vi "example-tx-c_api.vi"() -> ()   [LabVIEW 2024]
uses:
  <vilib>/Analysis/1siggen.llb/Ramp Pattern by Samples.vi
  uhd (generated from wizard into user.lib - manually fixed for rx example)/uhd.lvlib
  <vilib>/Analysis/NI_AALBase.lvlib
panel:
  out "ant_out out":string
  in  "stop":bool
  out "freq_out out":dbl
  in  "target_freq":dbl=1000000000.0 format="%#_6p"
  in  "ant":string="TX/RX"
  out "gain_out out":dbl
  in  "gain":dbl
  out "rate_out out":dbl
  in  "rate":dbl=1000000.0
  in  "chan":u64
  out "error out":errorcluster
  in  "args":string="type=b200"
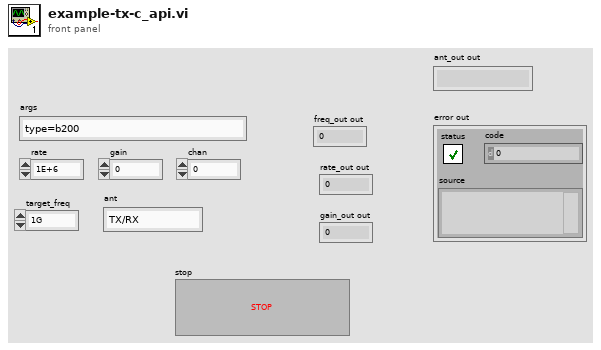
[diagram p1: front panel]
types:
  T1 = cluster{"cpu_format":string, "otw_format":string, "args":string, "channel_list":u64[], "n_channels":u64}
  T2 = cluster{"target_freq":dbl, "rf_freq_policy":u32, "@dummy control@":i8, "@dummy control@":i8, "@dummy control@":i8, "@dummy control@":i8, "rf_freq":dbl, "dsp_freq_policy":u32, "@dummy control@":i8, "@dummy control@":i8, "@dummy control@":i8, "@dummy control@":i8, "dsp_freq":dbl, "args":u64}
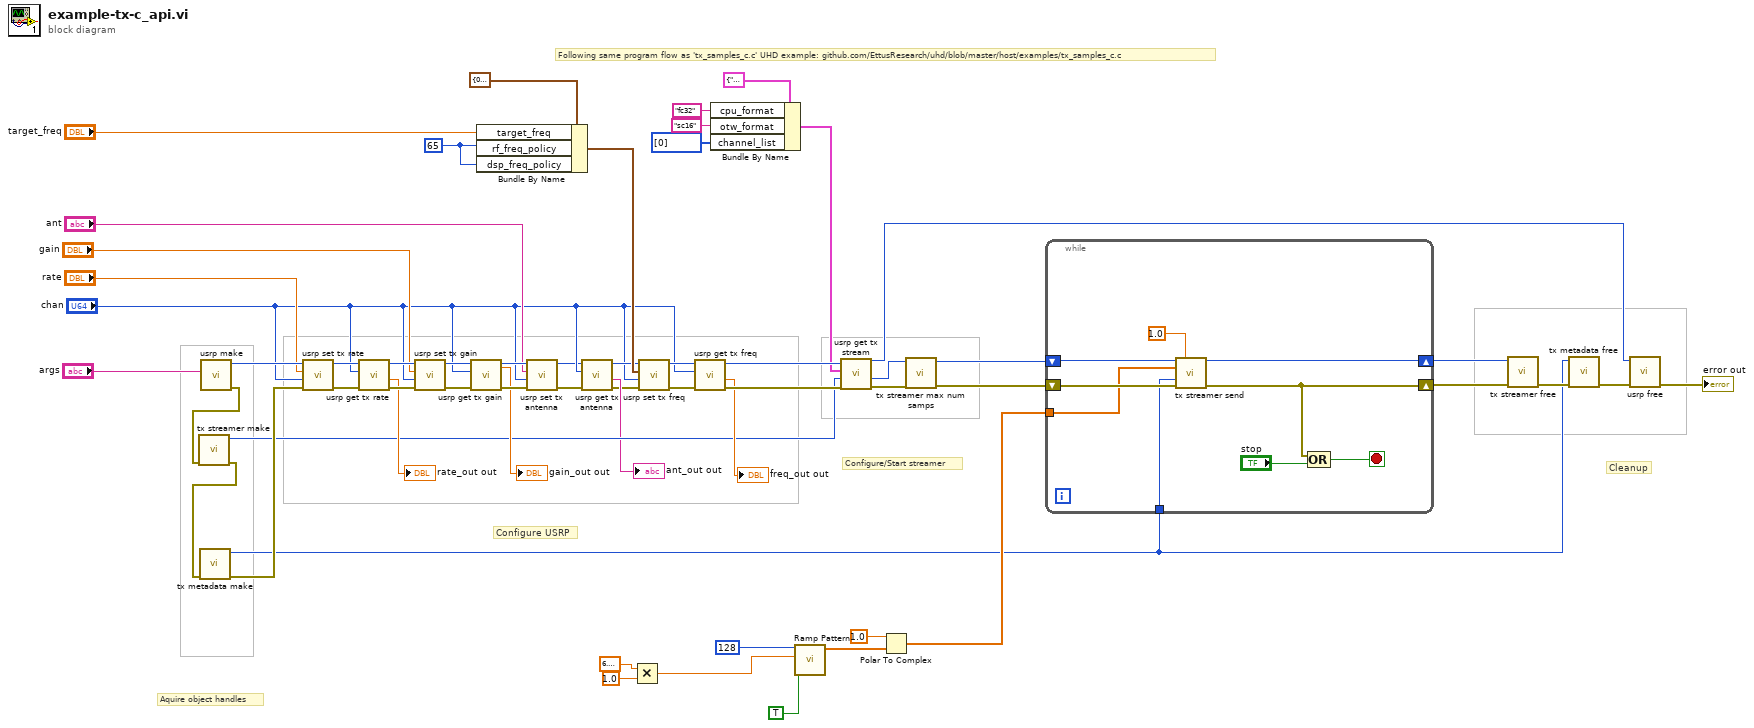
[diagram p0: block diagram]
diagram:
  w16 = u32 65 ("rf_freq_policy")
  # "Cleanup"
  # "Configure/Start streamer"
  # "Configure USRP"
  # "Aquire object handles"
  # "Following same program flow as 'tx_samples_c.c' UHD example: github.com/EttusResearch/uhd/blob/master/host/examples/tx_samples_c.c"
  n1 = call "usrp make.vi"("args"="args") -> ("error out"=w58:errorcluster, "h"=w56:u64)  [unwired: 8 in, 1 out]
  n2 = call "tx streamer make.vi"("error in (no error)"=w58) -> ("error out"=w42:errorcluster, "h out"=w13:u64)  [unwired: 8 in, 1 out]
  n3 = call "tx metadata make.vi"("error in (no error)"=w42) -> ("error out"=w55:errorcluster, "handle out"=w7:u64)  [unwired: 8 in, 1 out]
  n4 = call "usrp set tx rate.vi"("error in (no error)"=w55, "chan"="chan", "rate"="rate", "h"=w56) -> ("error out"=w54:errorcluster, "h 2"=w41:u64)  [unwired: 5 in, 1 out]
  n5 = call "usrp get tx rate.vi"("error in (no error)"=w54, "chan"="chan", "h"=w41) -> ("error out"=w53:errorcluster, "rate_out out"=→"rate_out out":dbl, "h 2"=w40:u64)  [unwired: 5 in, 1 out]
  n6 = call "usrp set tx gain.vi"("error in (no error)"=w53, "chan"="chan", "gain"="gain", "h"=w40) -> ("error out"=w52:errorcluster, "h 2"=w39:u64)  [unwired: 5 in, 1 out]
  n7 = call "usrp get tx gain.vi"("error in (no error)"=w52, "chan"="chan", "h"=w39) -> ("error out"=w51:errorcluster, "h 2"=w38:u64, "gain_out out"=→"gain_out out":dbl)  [unwired: 5 in, 1 out]
  n8 = Bundle By Name(cluster=T2 {"target_freq"=0.0, "rf_freq_policy"=78, "@dummy control@"=0, "@dummy control@"=0, "@dummy control@"=0, "@dummy control@"=0, "rf_freq"=0.0, "dsp_freq_policy"=78, "@dummy control@"=0, "@dummy control@"=0, "@dummy control@"=0, "@dummy control@"=0, "dsp_freq"=0.0, "args"=0} ("tune_request"), "target_freq"="target_freq", "rf_freq_policy"=w16, "dsp_freq_policy"=w16) -> (w15:T2)
  n9 = call "usrp set tx antenna.vi"("error in (no error)"=w51, "chan"="chan", "ant"="ant", "h"=w38) -> ("error out"=w3:errorcluster, "h 2"=w4:u64)  [unwired: 5 in, 1 out]
  n10 = call "usrp get tx antenna.vi"("error in (no error)"=w3, "chan"="chan", "h"=w4) -> ("error out"=w1:errorcluster, "ant_out out"=→"ant_out out":string, "h 2"=w6:u64)  [unwired: 5 in, 1 out]
  n11 = Multiply(x=6.283185307179586, y=1.0) -> (x*y=w27:dbl)
  n12 = call "usrp set tx freq.vi"("error in (no error)"=w1, "chan"="chan", "tune_request"=w15, "h"=w6) -> ("error out"=w50:errorcluster, "h 2"=w37:u64)  [unwired: 2 in, 4 out]
  n13 = call "usrp get tx freq.vi"("error in (no error)"=w50, "chan"="chan", "h"=w37) -> ("error out"=w49:errorcluster, "freq_out out"=→"freq_out out":dbl, "h 2"=w36:u64)  [unwired: 5 in, 1 out]
  n14 = Bundle By Name(cluster=T1 {"cpu_format"="", "otw_format"="", "args"="", "channel_list"=[], "n_channels"=0} ("stream_args 2"), "cpu_format"="fc32", "otw_format"="sc16", "channel_list"=u64[] [0]) -> (w8:T1)
  n15 = call-poly <vilib>:"Ramp Pattern.vi"("exclude end?"=TRUE, "end"=w27, "samples"=128) -> ("Ramp Pattern"=w31:dbl[])  [unwired: 7 in, 1 out]
  n16 = call "usrp get tx stream.vi"("error in (no error)"=w49, "h_out"=w13, "stream_args 2"=w8, "h"=w36) -> ("error out"=w48:errorcluster, "h_out 2"=w35:u64, "h 2"=w34:u64)  [unwired: 3 in, 2 out]
  n17 = Polar To Complex(1:w31, 2:1.0 ("r")) -> (0:w24:cdb[])
  n18 = call "tx streamer max num samps.vi"("error in (no error)"=w48, "h"=w35) -> ("error out"=w47:errorcluster, "h 2"=w33:u64)  [unwired: 6 in, 2 out]
  n19 = while {
    shift-right: [w65] -> w32
    shift-left: w33 -> [w66]
    shift-right: [w60] -> w44
    shift-left: w47 -> [w67]
    tunnel: w24 -> [w64]
    tunnel: w7 -> [w62]
    stop <- w59 stop-if-true
    n20 = call "tx streamer send.vi"("h"=w66, "timeout"=1.0, "buffs"=w64, "md"=w62, "error in (no error)"=w67) -> ("h 2"=w65:u64, "error out"=w60:errorcluster)  [unwired: 5 in, 4 out]
    n21 = Compound Arithmetic op=OR(w60, "stop") -> (w59:bool)
  }
  n22 = call "tx streamer free.vi"("error in (no error)"=w44, "h"=w32) -> ("error out"=w45:errorcluster)  [unwired: 7 in, 2 out]
  n23 = call "tx metadata free.vi"("error in (no error)"=w45, "handle"=w7) -> ("error out"=w46:errorcluster)  [unwired: 7 in, 2 out]
  n24 = call "usrp free.vi"("error in (no error)"=w46, "h"=w34) -> ("error out"=→"error out":errorcluster)  [unwired: 7 in, 2 out]
